vi "Build Shared Library Search Path.vi"(8 "Error In":errorcluster, 11 "lv-libssh2 Shared Library":path=path "") -> (0 "Error Out":errorcluster, 3 "Search Path":path[](array[path]))   [LabVIEW 2018, in "Toolkit.lvlib" / "SSH.lvclass"]
uses:
  SSH.lvclass
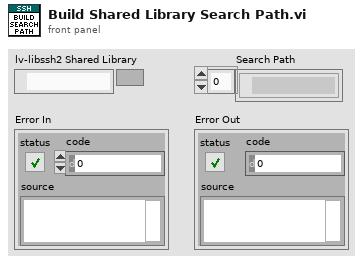
[diagram p1: front panel]
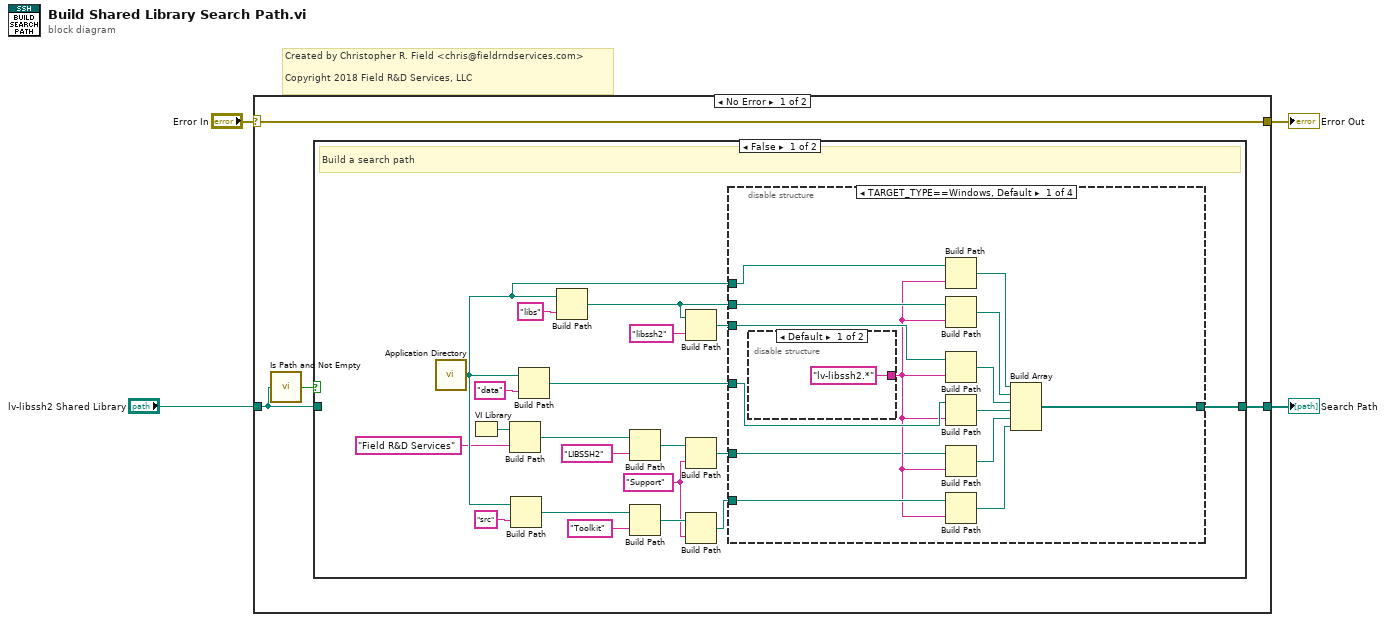
[diagram p0: block diagram]
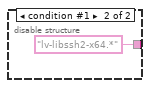
[diagram p2: hidden frame]
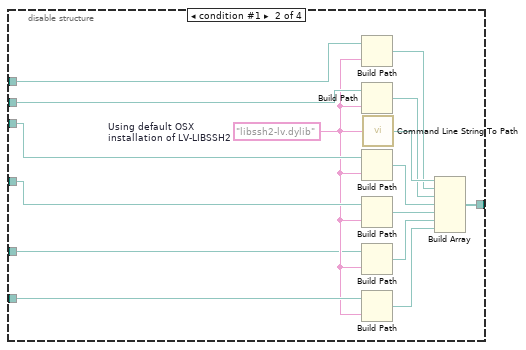
[diagram p3: hidden frame]
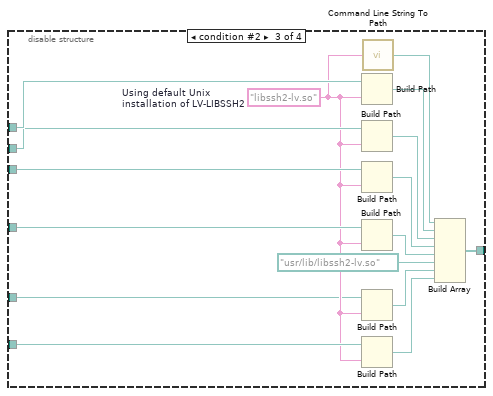
[diagram p4: hidden frame]
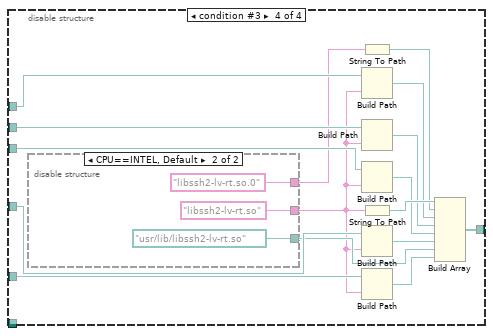
[diagram p5: hidden frame]
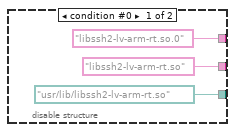
[diagram p6: hidden frame]
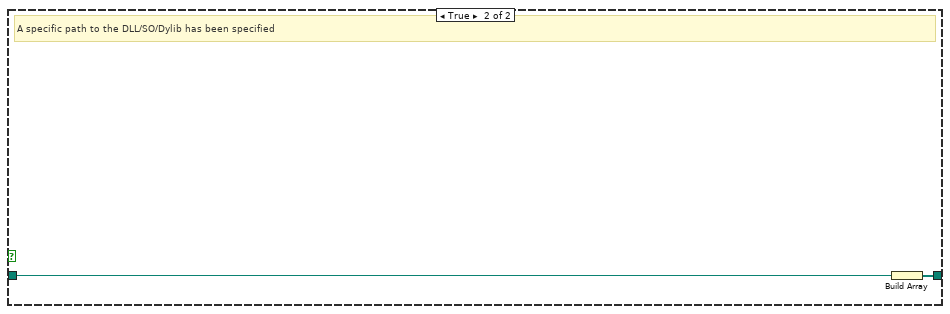
[diagram p7: hidden frame]
diagram:
  # "Created by Christopher R. Field <chris@fieldrndservices.com>\n\nCopyright 2018 Field R&D Services, LLC"
  n1 = case shown="No Error" "Error In" {
    selector: "Error In" -> [w5 w100]
    tunnel: [w8 _] -> w4
    tunnel: "lv-libssh2 Shared Library" -> [w7 _]
    tunnel: [w5 w100] -> w1
    frame No Error {
      n2 = call <vilib>:"Is Path and Not Empty.vi"("path"=w7) -> ("Is Path and Not Empty?"=w6:bool)  [unwired: 4 in]
      n3 = case shown="False" w6 {
        tunnel: w7 -> [_ w99]
        tunnel: [w24 w98] -> w8
        frame False {
          w11 = "Support" ("name or relative path")
          # "Build a search path"
          n4 = call <vilib>:"Application Directory.vi"() -> ("Application Directory"=w22:path)
          n5 = VI Library() -> (path=w16:path)
          n6 = Build Path(base path=w16, name or relative path="Field R&D Services") -> (appended path=w14:path)
          n7 = Build Path ("EXE include\nlocation")(base path=w22, name or relative path="src") -> (appended path=w27:path)
          n8 = Build Path ("EXE include\nlocation")(base path=w22, name or relative path="data") -> (appended path=w20:path)
          n9 = Build Path ("EXE include\nlocation")(base path=w22, name or relative path="libs") -> (appended path=w19:path)
          n10 = Build Path(base path=w14, name or relative path="LIBSSH2") -> (appended path=w13:path)
          n11 = Build Path ("EXE include\nlocation")(base path=w27, name or relative path="Toolkit") -> (appended path=w28:path)
          n12 = Build Path ("EXE include\nlocation")(base path=w19, name or relative path="libssh2") -> (appended path=w17:path)
          n13 = Build Path(base path=w13, name or relative path=w11) -> (appended path=w12:path)
          n14 = Build Path ("EXE include\nlocation")(base path=w28, name or relative path=w11) -> (appended path=w25:path)
          n15 = disable-structure shown="TARGET_TYPE==Windows, Default" {
            disable-tunnel: [w41 w58 w74 w91] -> w24
            disable-tunnel: w25 -> [w42 w57 w73 _]
            disable-tunnel: w22 -> [w40 w56 w67 w84]
            disable-tunnel: w19 -> [w39 w55 w66 w83]
            disable-tunnel: w20 -> [w38 w53 w64 w81]
            disable-tunnel: w17 -> [w37 w54 w65 w82]
            disable-tunnel: w12 -> [w35 w47 w62 w78]
            frame condition #0 (active) {
              n16 = disable-structure shown="Default" {
                disable-tunnel: ["lv-libssh2.*" ("name or relative path") "lv-libssh2-x64.*" ("name or relative path")] -> w36
                frame condition #0 (active) {
                }
                frame condition #1 {
                }
              }
              n17 = Build Path ("EXE include\nlocation")(base path=w40, name or relative path=w36) -> (appended path=w29:path)
              n18 = Build Path ("EXE include\nlocation")(base path=w39, name or relative path=w36) -> (appended path=w30:path)
              n19 = Build Path ("EXE include\nlocation")(base path=w37, name or relative path=w36) -> (appended path=w31:path)
              n20 = Build Path ("EXE include\nlocation")(base path=w38, name or relative path=w36) -> (appended path=w32:path)
              n21 = Build Path ("EXE include\nlocation")(base path=w35, name or relative path=w36) -> (appended path=w34:path)
              n22 = Build Path ("EXE include\nlocation")(base path=w42, name or relative path=w36) -> (appended path=w33:path)
              n23 = Build Array(w29, w30, w31, w32, w34, w33) -> (w41:path[])
            }
            frame condition #1 {
              w48 = "libssh2-lv.dylib"  # Using default OSX installation of LV-LIBSSH2
              n24 = Build Path ("EXE include\nlocation")(base path=w56, name or relative path=w48) -> (appended path=w52:path)
              n25 = Build Path ("EXE include\nlocation")(base path=w55, name or relative path=w48) -> (appended path=w51:path)
              n26 = Build Path ("EXE include\nlocation")(base path=w54, name or relative path=w48) -> (appended path=w50:path)
              n27 = Build Path ("EXE include\nlocation")(base path=w53, name or relative path=w48) -> (appended path=w49:path)
              n28 = Build Path ("EXE include\nlocation")(base path=w47, name or relative path=w48) -> (appended path=w46:path)
              n29 = Build Path ("EXE include\nlocation")(base path=w57, name or relative path=w48) -> (appended path=w45:path)
              n30 = call <vilib>:"Command Line String To Path.vi"("string"=w48) -> ("path"=w59:path)
              n31 = Build Array(w59, w52, w51, w50, w49, w46, w45) -> (w58:path[])
            }
            frame condition #2 {
              w63 = "libssh2-lv.so"  # Using default Unix installation of LV-LIBSSH2
              n32 = Build Path ("EXE include\nlocation")(base path=w67, name or relative path=w63) -> (appended path=w71:path)
              n33 = Build Path ("EXE include\nlocation")(base path=w66, name or relative path=w63) -> (appended path=w70:path)
              n34 = Build Path ("EXE include\nlocation")(base path=w65, name or relative path=w63) -> (appended path=w69:path)
              n35 = Build Path ("EXE include\nlocation")(base path=w64, name or relative path=w63) -> (appended path=w68:path)
              n36 = Build Path ("EXE include\nlocation")(base path=w62, name or relative path=w63) -> (appended path=w61:path)
              n37 = Build Path ("EXE include\nlocation")(base path=w73, name or relative path=w63) -> (appended path=w60:path)
              n38 = call <vilib>:"Command Line String To Path.vi"("string"=w63) -> ("path"=w75:path)
              n39 = Build Array(w75, w71, w70, w69, w68, path "/usr/lib/libssh2-lv.so" ("path"), w61, w60) -> (w74:path[])
            }
            frame condition #3 {
              n40 = disable-structure shown="CPU==INTEL, Default" {
                disable-tunnel: ["libssh2-lv-arm-rt.so.0" "libssh2-lv-rt.so.0"] -> w80
                disable-tunnel: ["libssh2-lv-arm-rt.so" "libssh2-lv-rt.so"] -> w77
                disable-tunnel: [path "/usr/lib/libssh2-lv-arm-rt.so" ("path") path "/usr/lib/libssh2-lv-rt.so" ("path")] -> w79
                frame condition #0 {
                }
                frame condition #1 (active) {
                }
              }
              n41 = String To Path(string=w80) -> (path=w89:path)
              n42 = Build Path ("EXE include\nlocation")(base path=w84, name or relative path=w77) -> (appended path=w85:path)
              n43 = Build Path ("EXE include\nlocation")(base path=w83, name or relative path=w77) -> (appended path=w88:path)
              n44 = Build Path ("EXE include\nlocation")(base path=w82, name or relative path=w77) -> (appended path=w87:path)
              n45 = String To Path(string=w77) -> (path=w90:path)
              n46 = Build Path ("EXE include\nlocation")(base path=w81, name or relative path=w77) -> (appended path=w86:path)
              n47 = Build Path ("EXE include\nlocation")(base path=w78, name or relative path=w77) -> (appended path=w76:path)
              n48 = Build Array(w90, w89, w85, w88, w87, w86, w79, w76) -> (w91:path[])
            }
          }
        }
        frame True {
          # "A specific path to the DLL/SO/Dylib has been specified"
          n49 = Build Array(w99) -> (w98:path[])
        }
      }
    }
    frame Error {
    }
  }
  "Search Path" <- w4
  "Error Out" <- w1
